vi "PathConfigurations.vi"() -> (0 "OhanaOS Path":path)   [LabVIEW 2009]
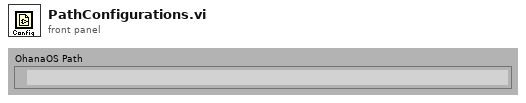
[diagram p1: front panel]
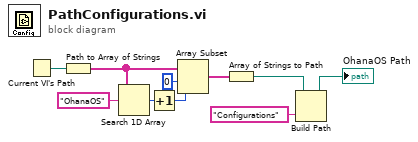
[diagram p0: block diagram]
diagram:
  n1 = Current VI's Path() -> (path=w10:path)
  n2 = Path to Array of Strings(0:w10) -> (2:w8:string[])  [unwired: 1 out]
  n3 = Search 1D Array(1D array=w8, element="OhanaOS" ("élément")) -> (index of element=w7:i32)  [unwired: 1 out]
  n4 = Increment(x=w7) -> (x+1=w4:i32)
  n5 = Array Subset(array=w8, index=0 ("Indice du tableau"), length=w4) -> (w5:string[])
  n6 = Array of Strings to Path(0:w5) -> (2:w3:path)  [unwired: 1 out]
  n7 = Build Path(base path=w3, name or relative path="Configurations" ("nom ou chemin relatif")) -> (appended path=→"OhanaOS Path":path)
